vi "Auto Shift Test.vi"() -> ()   [LabVIEW 2012]
uses:
  Encoder Values.ctl
  Auto Shift Settings.ctl
panel:
  in  "Right Encoder":dbl(slide) scale=0.0..20.0
  in  "Left Encoder":dbl(slide) scale=0.0..20.0
  in  "Right Motor":dbl(slide) scale=-1.0..1.0
  in  "Left Motor":dbl(slide) scale=-1.0..1.0
  in  "Auto Shift Settings":T1={"Enabled"=FALSE, "Upshift Speed"=6.0, "Downshift Speed"=3.0, "Upshift Throttle"=0.6000000000000001, "Turn Power Diff"=0.7, "Motor Limit"=100.0, "Encoder Limit"=1500.0}
  in  "Encoder Values":T2
  in  "Drive Controls":T3
  in  "stop":bool
  # "Motor Power"
  # "Encoder Speed"
  # "(uses MAX value)"
  # "(uses MIN value)"
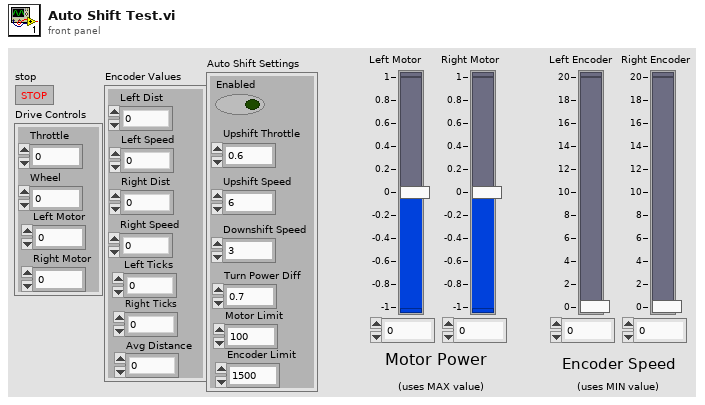
[diagram p1: front panel]
types:
  T1 = typedef "Auto Shift Settings.ctl" = cluster{"Enabled":bool, "Upshift Speed":dbl, "Downshift Speed":dbl, "Upshift Throttle":dbl, "Turn Power Diff":dbl, "Motor Limit":dbl, "Encoder Limit":dbl}
  T2 = typedef "Encoder Values.ctl" = cluster{"Left Dist":dbl, "Left Speed":dbl, "Right Dist":dbl, "Right Speed":dbl, "Left Ticks":dbl, "Right Ticks":dbl, "Avg Distance":dbl}
  T3 = cluster{"Throttle":dbl, "Wheel":dbl, "Right Motor":dbl, "Left Motor":dbl}
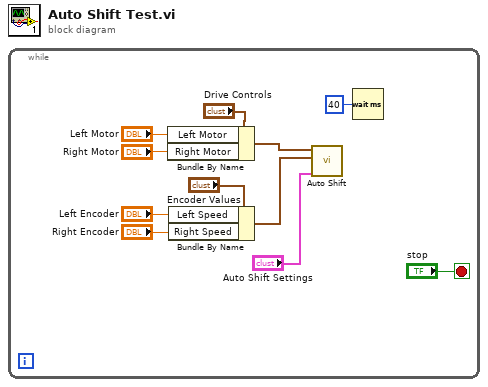
[diagram p0: block diagram]
diagram:
  n1 = while {
    stop <- "stop" stop-if-true
    n2 = Bundle By Name(cluster="Drive Controls", "Left Motor"="Left Motor", "Right Motor"="Right Motor") -> (w7:T3)
    n3 = Bundle By Name(cluster="Encoder Values", "Left Speed"="Left Encoder", "Right Speed"="Right Encoder") -> (w5:T2)
    n4 = call "Auto Shift.vi"("Auto Shift Settings"="Auto Shift Settings", "Encoder Values"=w5, "Drive Controls"=w7) -> ()  [unwired: 8 in, 1 out]
    n5 = Wait (ms)(milliseconds to wait=u32 40) -> ()  [unwired: 1 out]
  }
